vi "FTW-ActorConfig-FormatActorClassFilepath.vi"(0 "FTW Config String In":string="{}", 7 "Actor Instance":refnum<class "FTW-ActorInstance.lvclass">, 11 "error in":errorcluster) -> (4 "FTW Config String":string, 15 "error out":errorcluster)   [LabVIEW 2015]
uses:
  Instance/FTW-ActorInstance.lvclass
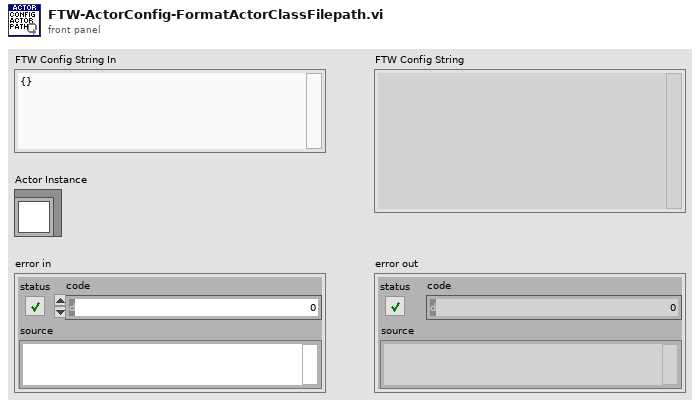
[diagram p1: front panel]
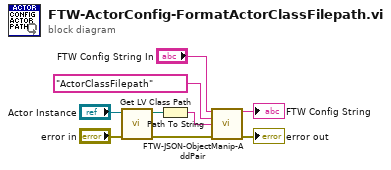
[diagram p0: block diagram]
diagram:
  n1 = call <vilib>:"Get LV Class Path.vi"("error in (no error)"="error in", "object"="Actor Instance") -> ("error out"=w3:errorcluster, "class path"=w2:path)  [unwired: 8 in]
  n2 = Path To String(path=w2) -> (string=w1:string)
  n3 = call "FTW-JSON-ObjectManip-AddPair.vi"("Input JSON Object"="FTW Config String In", "Key"="ActorClassFilepath", "Value"=w1, "error in"=w3) -> ("Output JSON Object"=→"FTW Config String":string, "error out"=→"error out":errorcluster)  [unwired: 10 in]
